vi "HEWH Read All MW100 Inputs.vi"(0 "MW100":refnum<visa-resource-name>="MW100", 2 "Semiphore":T1, 11 "Error In":errorcluster) -> (4 "dup VISA session":refnum<visa-resource-name>, 6 "All Data":dbl[](array[numeric]) format="%.4f", 15 "error out":errorcluster)   [LabVIEW 2012]
uses:
  ChannelSettings.ctl
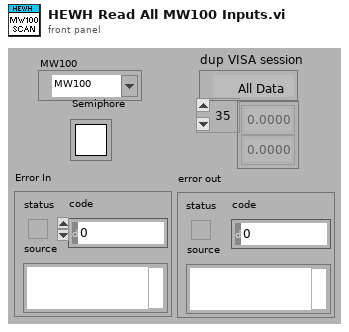
[diagram p1: front panel]
types:
  T1 = typedef "Semaphore RefNum" = refnum<k1>
  T2 = typedef "ChannelSettings.ctl" = u32
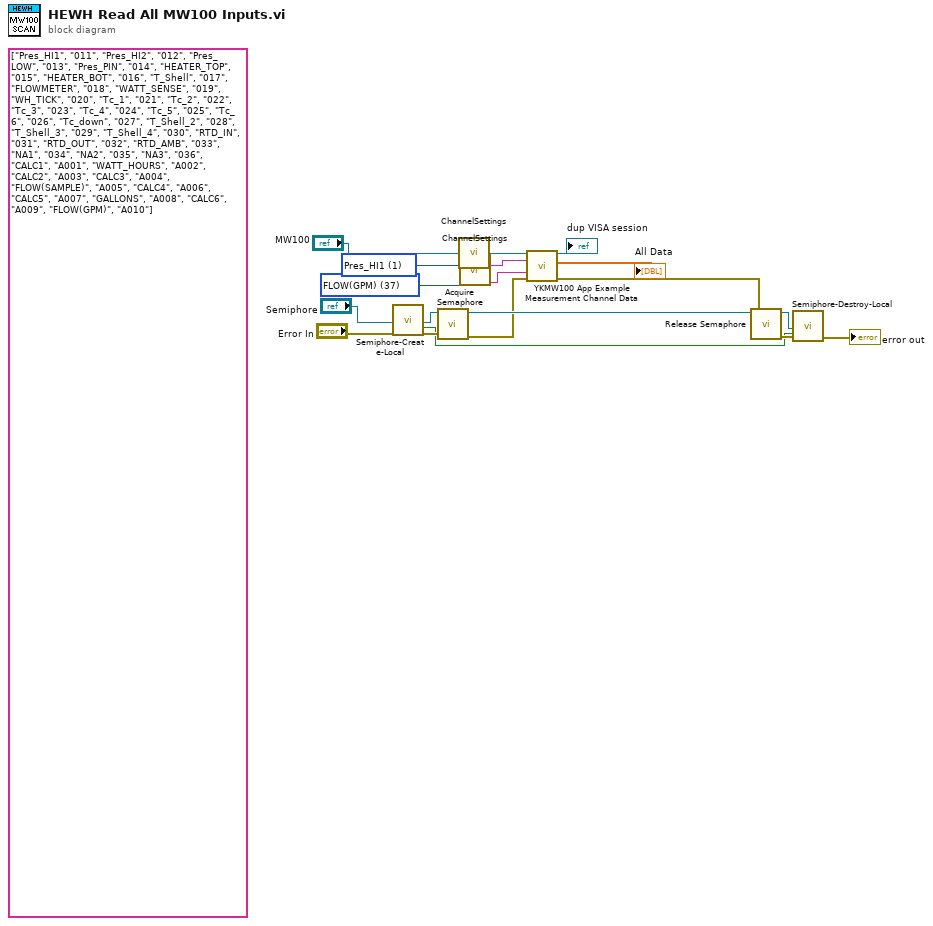
[diagram p0: block diagram]
diagram:
  (unwired) string[][] [["Pres_HI1", "011"], ["Pres_HI2", "012"], ["Pres_LOW", "013"], ["Pres_PIN", "014"], ["HEATER_TOP", "015"], ["HEATER_BOT", "016"], ["T_Shell", "017"], ["FLOWMETER", "018"], ["WATT_SENSE", "019"], ["WH_TICK", "020"], ["Tc_1", "021"], ["Tc_2", "022"], ["Tc_3", "023"], ["Tc_4", "024"], ["Tc_5", "025"], ["Tc_6", "026"], ["Tc_down", "027"], ["T_Shell_2", "028"], ["T_Shell_3", "029"], ["T_Shell_4", "030"], ["RTD_IN", "031"], ["RTD_OUT", "032"], ["RTD_AMB", "033"], ["NA1", "034"], ["NA2", "035"], ["NA3", "036"], ["CALC1", "A001"], ["WATT_HOURS", "A002"], ["CALC2", "A003"], ["CALC3", "A004"], ["FLOW(SAMPLE)", "A005"], ["CALC4", "A006"], ["CALC5", "A007"], ["GALLONS", "A008"], ["CALC6", "A009"], ["FLOW(GPM)", "A010"]] ("Sorted 2D Array")
  w12 = T2 37 items=["4-20_OUT", "Pres_HI1", "Pres_HI2", "Pres_LOW", "Pres_PIN", "HEATER_TOP", "HEATER_BOT", "T_Shell", "FLOWMETER", "WATT_SENSE", "WH_TICK", "Tc_1", "Tc_2", "Tc_3", "Tc_4", "Tc_5", "Tc_6", "Tc_down", "T_Shell_2", "T_Shell_3", "T_Shell_4", "RTD_IN", "RTD_OUT", "RTD_AMB", "INTF_TEMPFLO", "INTF_READY", "INTF_START", "INTF_STOP", "DRM_LOW", "DRM_HIGH", "PWR_MAIN", "VLV_DUMP", "VLV_OUT", "VLV_IN", "WATT_HOURS", "FLOW(SAMPLE)", "GALLONS", "FLOW(GPM)"] ("Channel_Enum")
  w13 = T2 1 items=["4-20_OUT", "Pres_HI1", "Pres_HI2", "Pres_LOW", "Pres_PIN", "HEATER_TOP", "HEATER_BOT", "T_Shell", "FLOWMETER", "WATT_SENSE", "WH_TICK", "Tc_1", "Tc_2", "Tc_3", "Tc_4", "Tc_5", "Tc_6", "Tc_down", "T_Shell_2", "T_Shell_3", "T_Shell_4", "RTD_IN", "RTD_OUT", "RTD_AMB", "INTF_TEMPFLO", "INTF_READY", "INTF_START", "INTF_STOP", "DRM_LOW", "DRM_HIGH", "PWR_MAIN", "VLV_DUMP", "VLV_OUT", "VLV_IN", "WATT_HOURS", "FLOW(SAMPLE)", "GALLONS", "FLOW(GPM)"] ("Channel_Enum")
  n1 = call "Semiphore-Create-Local.vi"("Semiphore"="Semiphore", "error in (no error)"="Error In") -> ("semaphore"=w8:T1, "Local?"=w5:bool, "error out"=w10:errorcluster)  [unwired: 15 in]
  n2 = call <vilib>:"Acquire Semaphore.vi"("error in (no error)"=w10, "semaphore"=w8) -> ("error out"=w1:errorcluster, "semaphore out"=w11:T1)  [unwired: 3 in, 1 out]
  n3 = call "ChannelSettings.vi"("Channel_Enum"=w13) -> ("Channel String"=w18:string)  [unwired: 10 in]
  n4 = call "ChannelSettings.vi"("Channel_Enum"=w12) -> ("Channel String"=w14:string)  [unwired: 10 in]
  n5 = call "YKMW100 App Example Measurement Channel Data.vi"("VISA session"="MW100", "Start Channel (001)"=w18, "End Channel (001)"=w14, "error in (no error)"=w1) -> ("dup VISA session"=→"dup VISA session":refnum<visa-resource-name>, "Data List"=→"All Data":dbl[], "error out"=w2:errorcluster)  [unwired: 4 in, 5 out]
  n6 = call <vilib>:"Release Semaphore.vi"("error in (no error)"=w2, "semaphore"=w11) -> ("error out"=w7:errorcluster, "semaphore out"=w6:T1)  [unwired: 4 in]
  n7 = call "Semiphore-Destroy-Local.vi"("Semiphore"=w6, "Local?"=w5, "error in (no error)"=w7) -> ("error out"=→"error out":errorcluster)  [unwired: 16 in]
